vi "grap display.vi"(8 "error in":errorcluster, 11 "file path (dialog if empty)":path) -> (0 "error out":errorcluster, 1 "HUMIDITY":string[](array[string]), 2 "AIR TEMPERATURE":string[](array[string]), 3 "XY GRAPH":cluster{"X":dbl[], "Y":dbl[]}[](array[cluster]))   [LabVIEW 2025]
uses:
  <vilib>/Utility/file.llb/Read Delimited Spreadsheet (string).vi
panel:
  out "XY Graph 2":cluster{"X":dbl[], "Y":dbl[]}[](graph)
  out "TEMP":string[](array[string])
  out "COF":string[](array[string])
  out "TIME":string[](array[string])
  out "all rows":string[][](array[string])
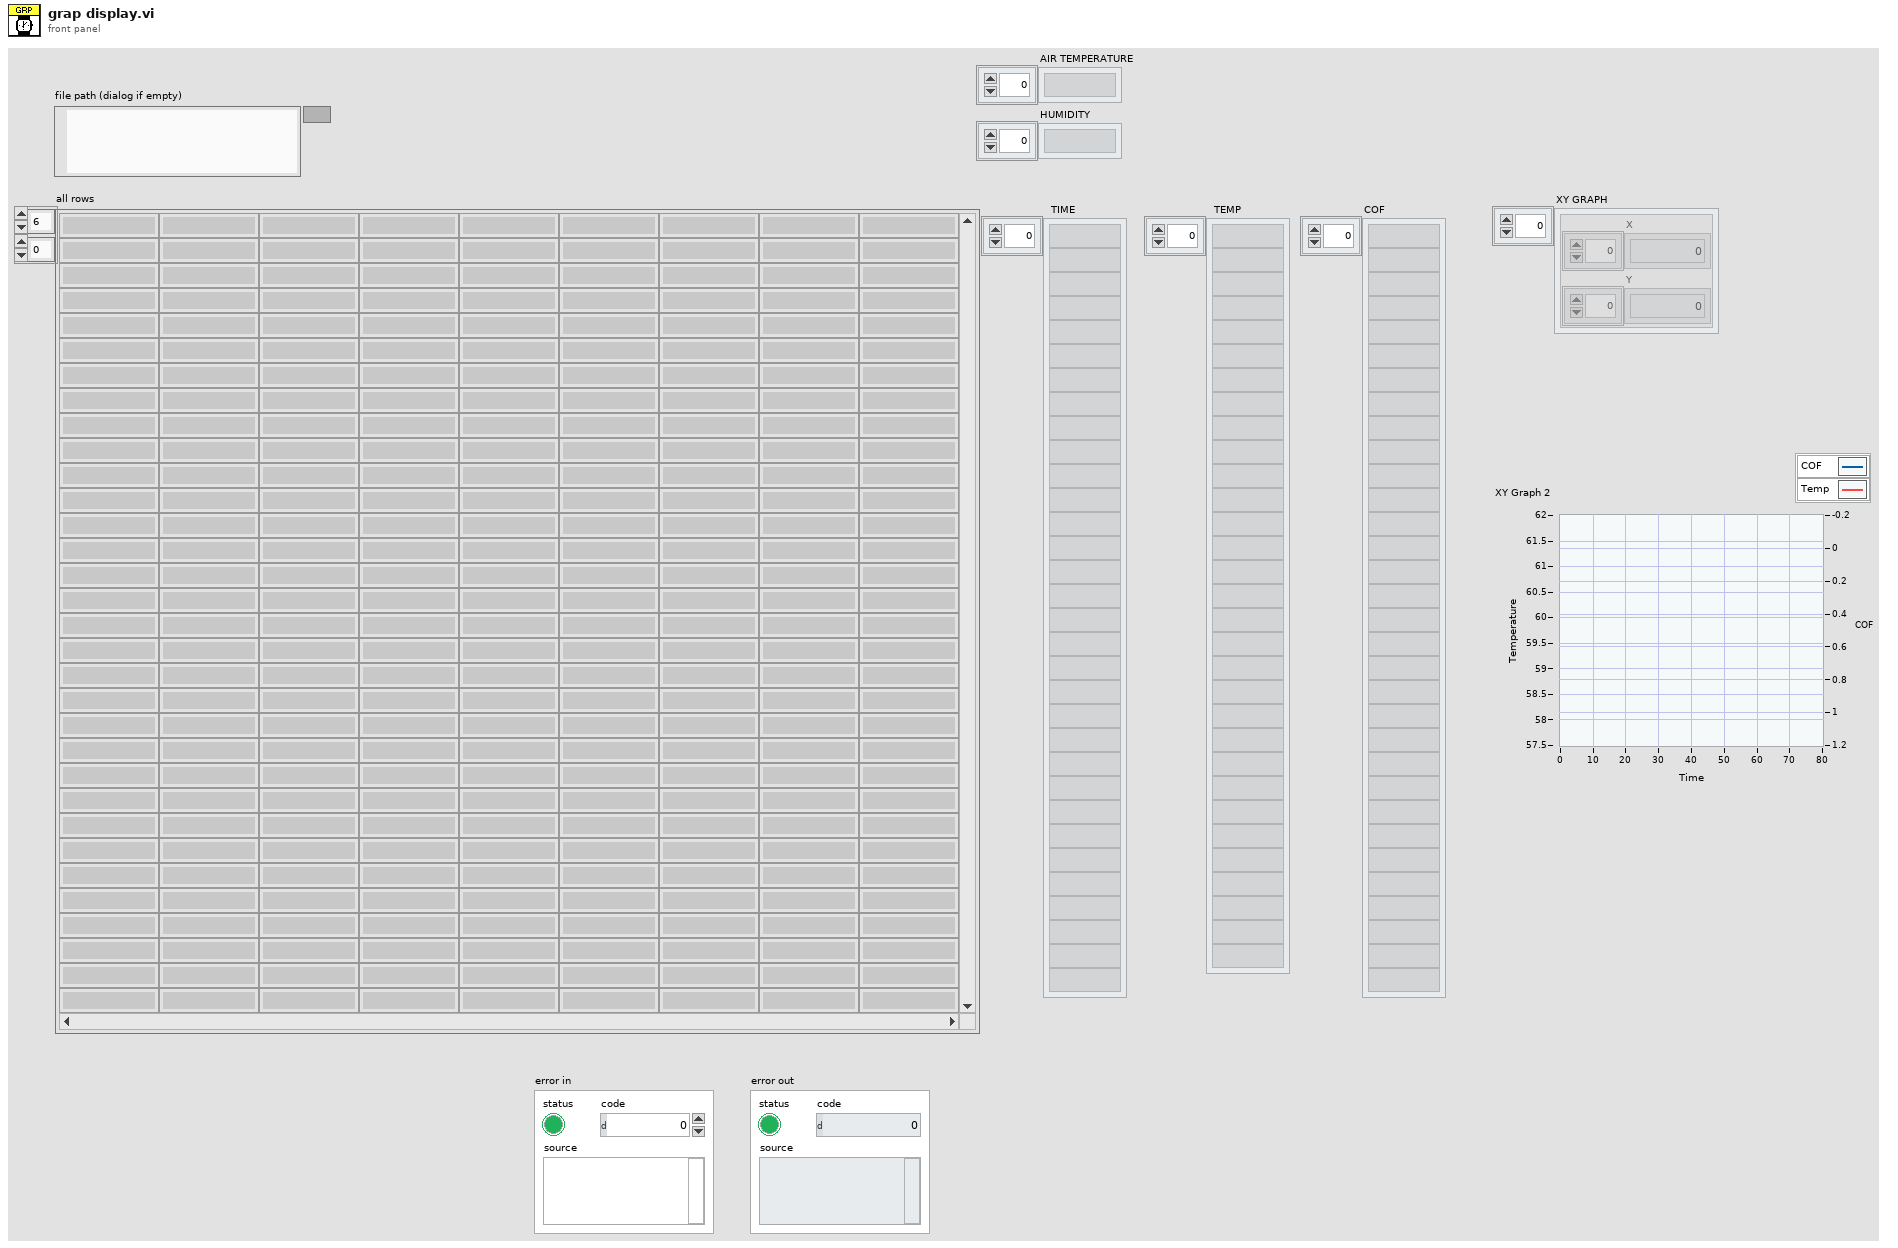
[diagram p1: front panel]
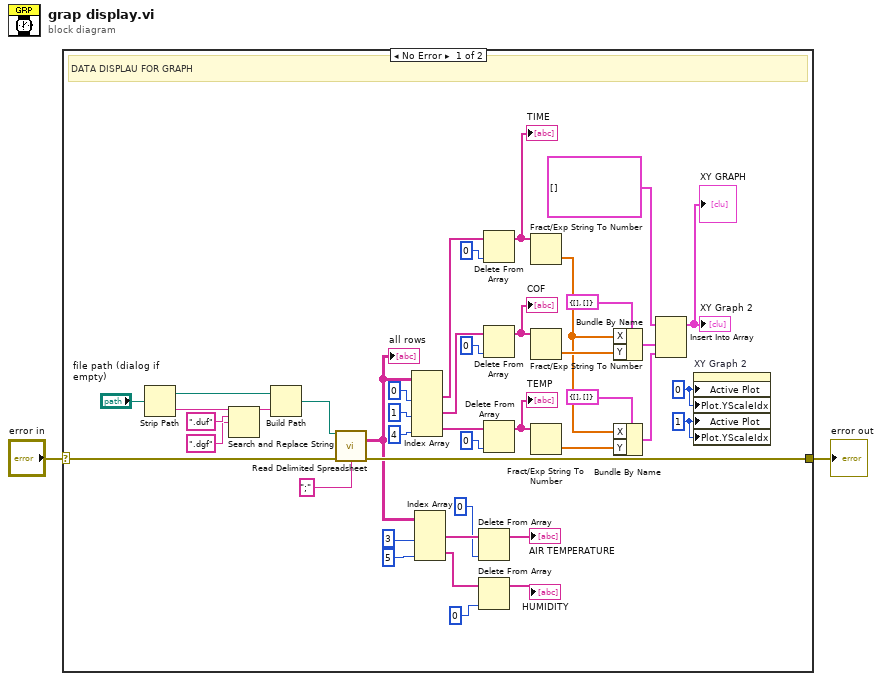
[diagram p0: block diagram]
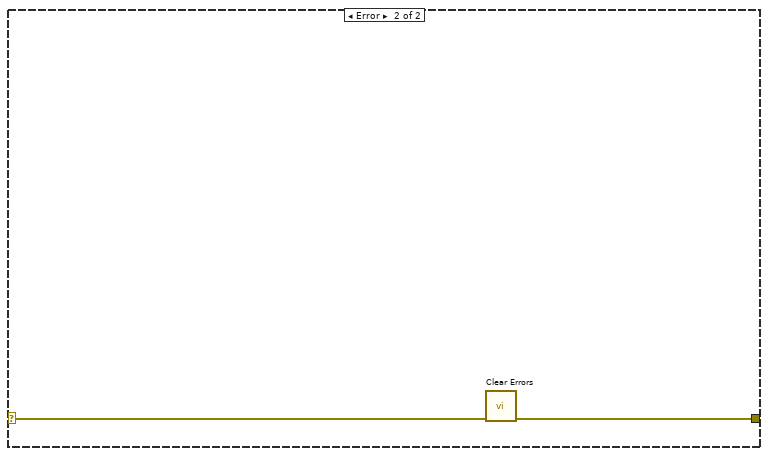
[diagram p2: hidden frame]
diagram:
  n1 = case shown="No Error" "error in" {
    selector: "error in" -> [w22 w46]
    tunnel: [w21 w45] -> w1
    frame No Error {
      w19 = u32 1 ("Active Plot")
      w20 = u32 0 ("Active Plot")
      # "DATA DISPLAU FOR GRAPH"
      n2 = Strip Path(path="file path (dialog if empty)") -> (stripped path=w4:path, name=w8:string)
      n3 = Search and Replace String(input string=w8, search string=".duf", replace string=".dgf" ("search string")) -> (result string=w5:string)  [unwired: 5 in, 3 out]
      n4 = Build Path(base path=w4, name or relative path=w5) -> (appended path=w3:path)
      n5 = call-poly <vilib>:"Read Delimited Spreadsheet.vi"("file path (dialog if empty)"=w3, "error in (no error)"=w22, "delimiter (\\t)"=";" ("delimiter (\\t)")) -> ("all rows"=w18:string[][], "error out"=w21:errorcluster)  [unwired: 7 in, 4 out]
      "all rows" <- w18
      n6 = Index Array(array=w18, index (col) #1=0 ("disabled index (col)"), index (col) #2=1 ("index (col)"), index (col) #3=4 ("index (col)")) -> (element #1=w32:string[], element #2=w26:string[], element #3=w31:string[])  [unwired: 3 in]
      n7 = Index Array(array=w18, index (col) #1=3 ("index (col)"), index (col) #2=5 ("index (col)")) -> (element #1=w15:string[], element #2=w14:string[])  [unwired: 2 in]
      n8 = Delete From Array(array=w15, index=0) -> (array with subset deleted=→"AIR TEMPERATURE":string[])  [unwired: 1 in, 1 out]
      n9 = Delete From Array(array=w14, index=0) -> (array with subset deleted=→"HUMIDITY":string[])  [unwired: 1 in, 1 out]
      n10 = Delete From Array(array=w32, index=0) -> (array with subset deleted=w27:string[])  [unwired: 1 in, 1 out]
      "TIME" <- w27
      n11 = Delete From Array(array=w26, index=0) -> (array with subset deleted=w25:string[])  [unwired: 1 in, 1 out]
      "COF" <- w25
      n12 = Delete From Array(array=w31, index=0) -> (array with subset deleted=w24:string[])  [unwired: 1 in, 1 out]
      "TEMP" <- w24
      n13 = Fract/Exp String To Number(string=w27) -> (number=w35:dbl[])  [unwired: 3 in, 1 out]
      n14 = Fract/Exp String To Number(string=w25) -> (number=w37:dbl[])  [unwired: 3 in, 1 out]
      n15 = Fract/Exp String To Number(string=w24) -> (number=w34:dbl[])  [unwired: 3 in, 1 out]
      n16 = Bundle By Name(cluster=cluster{"X":dbl[], "Y":dbl[]} {"X"=[], "Y"=[]} ("new element/subarray"), "X"=w35, "Y"=w37) -> (w39:cluster{"X":dbl[], "Y":dbl[]})
      n17 = Bundle By Name(cluster=cluster{"X":dbl[], "Y":dbl[]} {"X"=[], "Y"=[]} ("new element/subarray"), "X"=w35, "Y"=w34) -> (w33:cluster{"X":dbl[], "Y":dbl[]})
      n18 = Insert Into Array(array=cluster{"X":dbl[], "Y":dbl[]}[] [] ("XY Graph"), new element #1=w39, new element #2=w33) -> (→"XY Graph 2" →"XY GRAPH":cluster{"X":dbl[], "Y":dbl[]}[])  [unwired: 1 in]
      n19 = property on="XY Graph 2" class="XYGraph (strict)"("Active Plot"=w20, "Plot.YScaleIdx"=w20, "Active Plot"=w19, "Plot.YScaleIdx"=w19) -> ()  [unwired: 2 in, 2 out]
    }
    frame Error {
      n20 = call <vilib>:"Clear Errors.vi"("error in (no error)"=w46) -> ("error out"=w45:errorcluster)  [unwired: 5 in, 1 out]
    }
  }
  "error out" <- w1
